vi "Explorer Hat Pro Example.vi"() -> ()   [LabVIEW 2020]
uses:
  LINX-ADS1015/ADS1015 Sample Rate.ctl
  LINX-ADS1015/Programmable Gain Selection.ctl
  LINX-ExplorerHatPro/Output Pins.ctl
  LINX-ADS1015/Channel Selection.ctl
  <vilib>/MakerHub/LINX/Public/Utilities/Open Local.vi
  <vilib>/MakerHub/LINX/LMH-LINX.lvlib
  LINX-ExplorerHatPro/LINX-ExplorerHatPro.lvclass
  LINX-ADS1015/LINX-ADS1X15.lvclass
panel:
  out "ADC Values":dbl[](array[numeric])
  out "ADC Channels":dbl[][](graph)
  out "Error Out":errorcluster
  in  "Stop":bool
  in  "Output 4":bool
  in  "Output 3":bool
  in  "Output 2":bool
  in  "Output 1":bool
  in  "LED 4":bool
  in  "LED 3":bool
  in  "LED 2":bool
  in  "LED 1":bool
  out "Button 8":bool
  out "Button 7":bool
  out "Button 6":bool
  out "Button 5":bool
  out "Button 4":bool
  out "Button 3":bool
  out "Button 2":bool
  out "Button 1":bool
  # "Explorer Hat Pro Example"
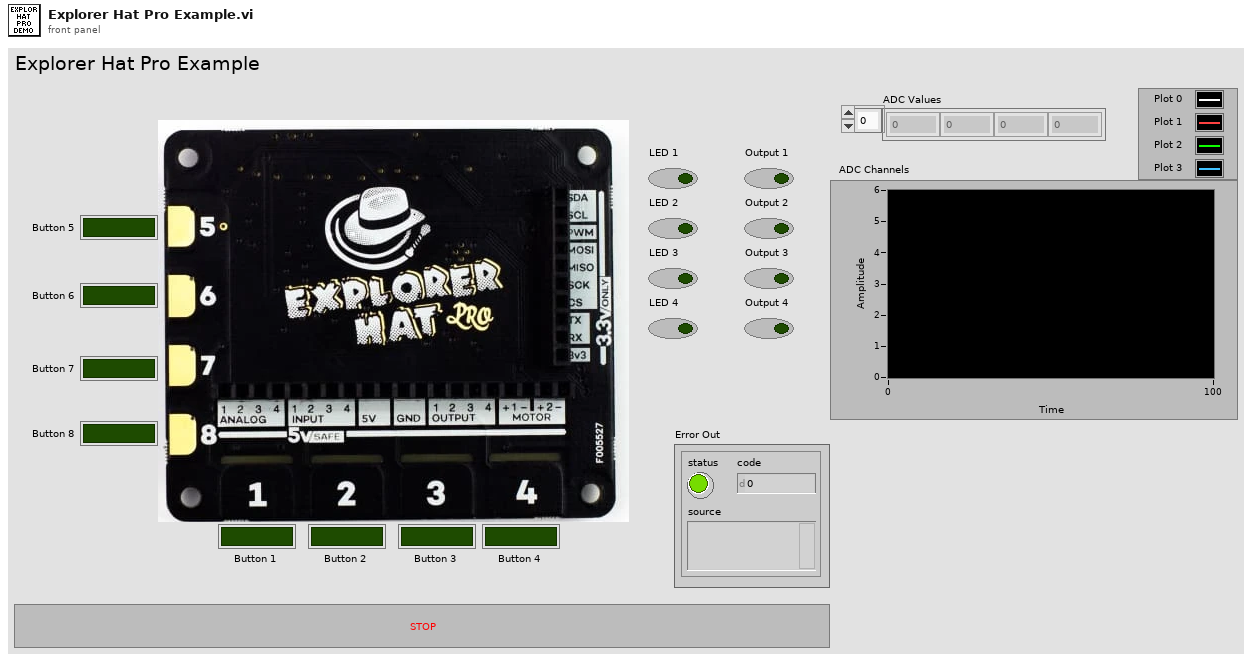
[diagram p1: front panel]
types:
  T1 = typedef "LINX-ADS1X15.lvclass/Programmable Gain Selection.ctl" = enum16{"+/-6.144V (2/3)", "+/-4.096V (1)", "+/-2.048V (2)", "+/-1.024V (4)", "+/-0.512V (8)", "+/-0.256V (16)"}
  T2 = typedef "LINX-ADS1X15.lvclass/ADS1015 Sample Rate.ctl" = u16
  T3 = typedef "LMH-LINX.lvlib/LINX Ref.ctl" = cluster{"IO":T4, "Interface":T5, "LINX Device Config":T6}
  T4 = typedef "LMH-LINX.lvlib/Platform.ctl" = enum16{"Remote", "Local"}
  T5 = typedef "LMH-LINX.lvlib/Interface.ctl" = enum16{"Serial", "TCP"}
  T6 = typedef "LMH-LINX.lvlib/Device.lvlib/LINX Device Config.ctl" = cluster{"Interface":T5, "COM Port":refnum<visa-resource-name>, "TCP Configuration":T7, "Device Family":u8, "Device ID":u8, "Device Name":string, "TCP Ref":refnum<k5>, "Channels":T8}
  T7 = typedef "LMH-LINX.lvlib/Device.lvlib/TCP Config.ctl" = cluster{"IP Address":string, "Port":u16}
  T8 = typedef "LMH-LINX.lvlib/Channels.ctl" = cluster{"DI":u8[], "DO":u8[], "AI":u8[], "AO":u8[], "PWM":u8[], "QE":u8[], "UART":u8[], "I2C 2":u8[], "SPI":u8[], "CAN":u8[], "Servo":u8[], "AI Ref (V)":dbl, "AI Resolution (Bits)":u8, "AO Ref (V)":dbl, "AO Resolution (Bits)":u8}
  T9 = typedef "LINX-ADS1X15.lvclass/Channel Selection.ctl" = enum16{"Differential 0-1", "Differential 2-3", "Single Ended 0", "Single Ended 1", "Single Ended 2", "Single Ended 3"}
  T10 = typedef "LINX-ExplorerHatPro.lvclass/Output Pins.ctl" = enum16{"LED1", "LED2", "LED3", "LED4", "OUTPUT1", "OUTPUT2", "OUTPUT3", "OUTPUT4"}
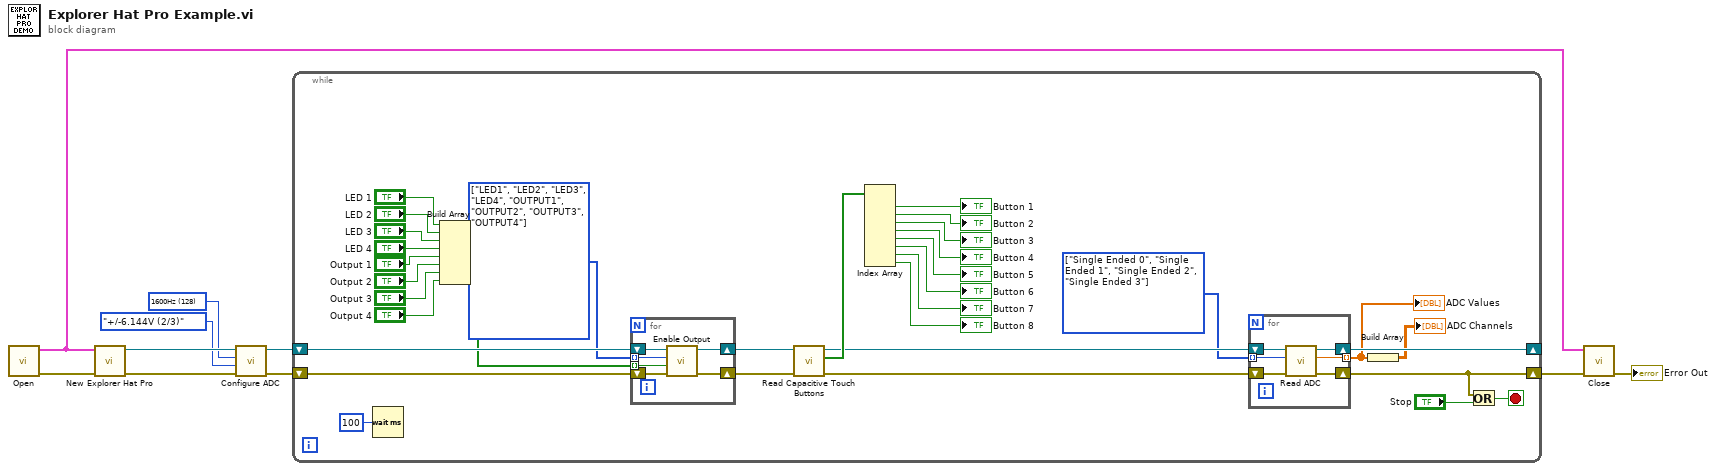
[diagram p0: block diagram]
diagram:
  w2 = T2 128 items=["128Hz"=0, "250Hz"=32, "490Hz"=64, "920Hz"=96, "1600Hz"=128, "2400Hz"=160, "3300Hz"=192] ("Sample Rate")
  n1 = call-poly <vilib>:"Open.vi"() -> ("Error Out"=w9:errorcluster, "LINX Resource"=w8:T3)  [unwired: 9 in, 1 out]
  n2 = call "New Explorer Hat Pro.vi"("error in (no error)"=w9, "LINX Resource"=w8) -> ("error out"=w5:errorcluster, "ExplorerHatPro out"=w6:refnum<class "LINX-ExplorerHatPro.lvclass">)  [unwired: 8 in]
  n3 = call "Configure ADC.vi"("error in (no error)"=w5, "Gain Values"=Programmable_Gain_Selection."+/-6.144V (2/3)", "Sample Rate"=w2, "ExplorerHatPro in"=w6) -> ("error out"=w4:errorcluster, "ExplorerHatPro out"=w3:refnum<class "LINX-ExplorerHatPro.lvclass">)  [unwired: 6 in]
  n4 = while {
    shift-right: [w15] -> w10
    shift-left: w4 -> [w43]
    shift-right: [w14] -> _
    shift-left: w3 -> [w42]
    stop <- w30 stop-if-true
    w13 = T9[] [enum."Single Ended 0", enum."Single Ended 1", enum."Single Ended 2", enum."Single Ended 3"] items=["Differential 0-1", "Differential 2-3", "Single Ended 0", "Single Ended 1", "Single Ended 2", "Single Ended 3"] ("Array")
    w32 = T10[] [enum."LED1", enum."LED2", enum."LED3", enum."LED4", enum."OUTPUT1", enum."OUTPUT2", enum."OUTPUT3", enum."OUTPUT4"] items=["LED1", "LED2", "LED3", "LED4", "OUTPUT1", "OUTPUT2", "OUTPUT3", "OUTPUT4"] ("Array")
    n5 = Wait (ms)(milliseconds to wait=u32 100) -> ()  [unwired: 1 out]
    n6 = Build Array("LED 1", "LED 2", "LED 3", "LED 4", "Output 1", "Output 2", "Output 3", "Output 4") -> (w33:bool[])
    n7 = for {
      shift-right: [w53] -> w28
      shift-left: w42 -> [w54]
      shift-right: [w52] -> w27
      shift-left: w43 -> [w55]
      tunnel: w33 -> [w51] mode=indexing
      tunnel: w32 -> [w50] mode=indexing
      n8 = call "Enable Output.vi"("error in (no error)"=w55, "Enable?"=w51, "Output"=w50, "LINX-ExplorerHatPro in"=w54) -> ("error out"=w52:errorcluster, "LINX-ExplorerHatPro out"=w53:refnum<class "LINX-ExplorerHatPro.lvclass">)  [unwired: 6 in]
    }
    n9 = call "Read Capacitive Touch Buttons.vi"("error in (no error)"=w27, "ExplorerHatPro in"=w28) -> ("error out"=w16:errorcluster, "Explorer Hat Buttons"=w26:bool[], "ExplorerHatPro out"=w17:refnum<class "LINX-ExplorerHatPro.lvclass">)  [unwired: 7 in]
    n10 = Index Array(array=w26) -> (element #1=→"Button 1":bool, element #2=→"Button 2":bool, element #3=→"Button 3":bool, element #4=→"Button 4":bool, element #5=→"Button 5":bool, element #6=→"Button 6":bool, element #7=→"Button 7":bool, element #8=→"Button 8":bool)  [unwired: 8 in]
    n11 = for {
      tunnel: w13 -> [w45] mode=indexing
      shift-right: [w46] -> w14
      shift-left: w17 -> [w49]
      shift-right: [w47] -> w15
      shift-left: w16 -> [w48]
      tunnel: [w44] -> w12 mode=indexing
      n12 = call "Read ADC.vi"("error in (no error)"=w48, "ADC Channel Selection"=w45, "ExplorerHatPro in"=w49) -> ("error out"=w47:errorcluster, "ADC Volts"=w44:dbl, "ExplorerHatPro out"=w46:refnum<class "LINX-ExplorerHatPro.lvclass">)  [unwired: 6 in]
    }
    "ADC Values" <- w12
    n13 = Build Array(w12) -> (→"ADC Channels":dbl[][])
    n14 = Or(x=w15, y="Stop") -> (x .or. y?=w30:bool)
  }
  n15 = call <vilib>:"Close.vi"("Error In"=w10, "LINX Resource"=w8) -> ("Error Out"=→"Error Out":errorcluster)  [unwired: 9 in]
